vi "Tell Child Init.vi"(4 "Alias":string, 7 "Actor in":refnum<class "Actor.lvclass">, 8 "Error in":errorcluster, 10 "Input":T1) -> (0 "Error out":errorcluster, 1 "Told":bool, 5 "Actor out":refnum<class "Actor.lvclass">)   [LabVIEW 2020, in "_Template.lvlib" / "Templates.lvlib" / "TEMPLATE jettl Msg.lvlib" / "TEMPLATE.lvlib"]
uses:
  TEMPLATE/TEMPLATE.lvlib
  TEMPLATE Msg/TEMPLATE Msg.lvclass
  TEMPLATE Msg Input/TEMPLATE Msg Input.lvclass
  TEMPLATE Msg Output/TEMPLATE Msg Output.lvclass
  jettl/jettl/jettl.lvlib
  Input.ctl
  TEMPLATE jettl Msg.lvlib
  Output.ctl
  jettl/jettl/Transport/Transport.lvclass
  jettl/jettl/Msg/Msg.lvclass
  jettl/jettl/Msgs.ctl
  jettl/jettl/Unified Layer.ctl
  jettl/jettl/Actor Attributes.ctl
  jettl/jettl/Relation.ctl
  jettl/jettl/Teller.ctl
  jettl/jettl/Msg Output/Msg Output.lvclass
  jettl/jettl/Msg Input/Msg Input.lvclass
  jettl/jettl/Msg Attributes.ctl
  jettl/jettl/Actor/Actor.lvclass
panel:
  # "This front panel should not be manipulated."
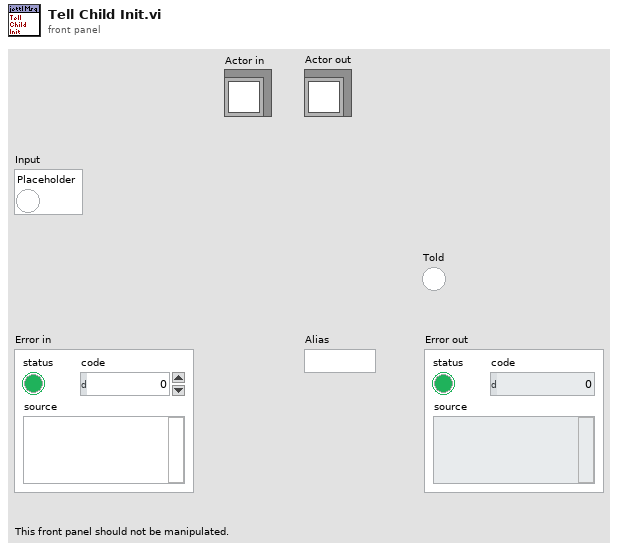
[diagram p1: front panel]
types:
  T1 = typedef "_Template.lvlib/Templates.lvlib/TEMPLATE jettl Msg.lvlib/Input.ctl" = cluster{"Placeholder":bool}
  T2 = typedef "_Template.lvlib/Templates.lvlib/TEMPLATE jettl Msg.lvlib/Output.ctl" = cluster{"Placeholder":bool}
  T3 = typedef "jettl.lvlib/Msg Attributes.ctl" = cluster{"Msg":refnum<class "Msg.lvclass">, "Msg Input":refnum<class "Msg Input.lvclass">, "Msg Output":refnum<class "Msg Output.lvclass">, "Teller":refnum<data-value>}
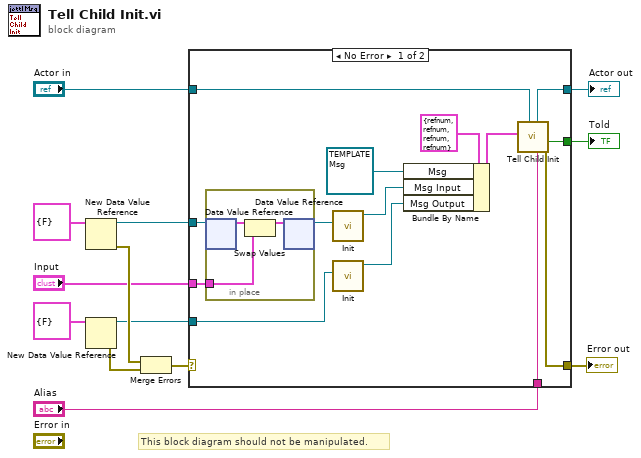
[diagram p0: block diagram]
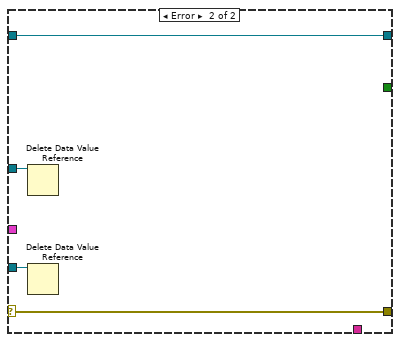
[diagram p2: hidden frame]
diagram:
  # "This block diagram should not be manipulated."
  n1 = New Data Value Reference(data value=T1 {"Placeholder"=FALSE} ("Input")) -> (data value reference=w13:refnum<data-value>, error out=w10:errorcluster)  [unwired: 1 in]
  n2 = New Data Value Reference(data value=T2 {"Placeholder"=FALSE} ("Output")) -> (data value reference=w8:refnum<data-value>, error out=w9:errorcluster)  [unwired: 1 in]
  n3 = Merge Errors(w10, w9) -> (w7:errorcluster)
  n4 = case shown="No Error" w7 {
    selector: w7 -> [_ w33]
    tunnel: w13 -> [w27 w34]
    tunnel: [w22 w33] -> w3
    tunnel: "Input" -> [w26 _]
    tunnel: w8 -> [w16 w32]
    tunnel: [w25 _] -> w6
    tunnel: [w24 w31] -> w5
    tunnel: "Actor in" -> [w23 w31]
    tunnel: "Alias" -> [w14 _]
    frame No Error {
      n5 = in-place {
        in-place-border: w26 -> [w29]
        n6 = in-place-dvr #1(w27) -> (w30:T1)  [unwired: 1 out]
        n7 = Swap Values(12:w30, 14:w29) -> (1:w28:T1)  [unwired: 1 in, 1 out]
        n8 = in-place-dvr #1(w28) -> (w17:refnum<data-value>)  [unwired: 1 out]
      }
      n9 = call "Init.vi"("Input"=w17) -> ("TEMPLATE Msg Input"=w20:refnum<class "TEMPLATE Msg Input.lvclass">)  [unwired: 10 in]
      n10 = call "Init.vi"("Output"=w16) -> ("TEMPLATE Msg Output"=w21:refnum<class "TEMPLATE Msg Output.lvclass">)  [unwired: 10 in]
      n11 = Bundle By Name(cluster=T3 {"Msg"=refnum, "Msg Input"=refnum, "Msg Output"=refnum, "Teller"=refnum} ("Msg Attributes"), "Msg"=refnum<class "TEMPLATE Msg.lvclass"> refnum ("_Template.lvlib:Templates.lvlib:TEMPLATE jettl Msg.lvlib:TEMPLATE Msg.lvlib:TEMPLATE Msg.lvclass"), "Msg Input"=w20, "Msg Output"=w21) -> (w15:T3)
      n12 = call "Tell Child Init.vi"("Alias"=w14, "Actor in"=w23, "Msg Attributes"=w15) -> ("Error out"=w22:errorcluster, "Told"=w25:bool, "Actor out"=w24:refnum<class "Actor.lvclass">)  [unwired: 6 in]
    }
    frame Error {
      n13 = Delete Data Value Reference(data value reference=w34) -> ()  [unwired: 1 in, 2 out]
      n14 = Delete Data Value Reference(data value reference=w32) -> ()  [unwired: 1 in, 2 out]
    }
  }
  "Error out" <- w3
  "Actor out" <- w5
  "Told" <- w6
